vi "ECS-1408-FPGA2-EPTx.vi"() -> ()   [LabVIEW 2015, in "ECS-FPGA.lvlib"]
uses:
  ECS-FPGA.lvlib
  <vilib>/Powertrain Controls/Device Drivers/Engine Position Tracking/EPTx/RevA/FPGA/Controls/EPTxSupervisor.ctl
  <vilib>/Powertrain Controls/Device Drivers/Engine Position Tracking/EPTx/RevA/FPGA/Controls/EPTxFuelSparkControl.ctl
  <vilib>/Powertrain Controls/Device Drivers/Engine Position Tracking/EPTx/RevA/FPGA/Controls/EPTxControl.ctl
  <vilib>/Powertrain Controls/Device Drivers/Engine Position Tracking/EPTx/RevA/FPGA/Controls/EPTxConfig.ctl
  <vilib>/Powertrain Controls/Device Drivers/Engine Position Tracking/EPTx/RevA/FPGA/Controls/EPTxTooth.ctl
  <vilib>/Platform/TimedLoop/XDataNode/timing_clust.ctl
  <vilib>/Platform/TimedLoop/XDataNode/nitl_modes.ctl
  <vilib>/Platform/TimedLoop/XDataNode/wakeup.ctl
  <vilib>/Powertrain Controls/Device Drivers/Engine Position Tracking/EPTx/RevA/FPGA/Controls/EPTxSignals.ctl
  <vilib>/rvi/Emulation/niFpgaGetClockAttributes.vi
  <vilib>/rvi/Emulation/niFpgaSctlEmulationGetInTimedLoop.vi
  <vilib>/rvi/Emulation/niFpgaEmulationReportErrorSimple.vi
  <vilib>/rvi/eio/common/nirviEmuTemplateMethod_errors.vi
  <vilib>/rvi/Emulation/niFpgaCriticalErrorInLSC.vi
  <vilib>/eio/EIONode/EIONode.xnode
  <vilib>/Platform/TimedLoop/XDataNode/XDataNode.xnode
  <vilib>/Platform/TimedLoop/XDataNode/XDNodeRunTimeDep.lvlib
  <vilib>/Powertrain Controls/Device Drivers/Engine Position Tracking/EPTx/RevA/FPGA/EPTx - RevA - FPGA.lvlib
panel:
  in  "DI-4.PlsGen_Config_Channel3":T1
  in  "DI-4.PlsGen_Config_Channel2":T1
  in  "DI-4.PlsGen_Config_Channel1":T1
  in  "DI-3.PlsGen_Config_Channel3":T1
  in  "DI-3.PlsGen_Config_Channel2":T1
  in  "DI-3.PlsGen_Config_Channel1":T1
  in  "DI-2.PlsGen_Config_Channel3":T1
  in  "DI-2.PlsGen_Config_Channel2":T1
  in  "DI-2.PlsGen_Config_Channel1":T1
  out "EPTxTooth":T2
  in  "EPTxConfig":T3
  in  "EPTxControl":T4
  in  "9269-1.AO3":fxp<+/-,20,5> format="%.17g"
  in  "9269-1.AO2":fxp<+/-,20,5> format="%.17g"
  in  "9269-1.AO1":fxp<+/-,20,5> format="%.17g"
  in  "9269-1.AO0":fxp<+/-,20,5> format="%.17g"
  in  "ESTTL-1.Sequences":T5(array[cluster])
  in  "ESTTL-1.Config":T6
  in  "DI-4.Control":T7 caption="DIControl"
  in  "DI-4.IPhaseInterface":T8(array[cluster]) caption="IPhaseInterface"
  in  "DI-4.ScopeRead":bool caption="DIScopeRead"
  out "DI-4.ScopeData":T9 caption="DIScopeData"
  out "DI-4.Data":T10 caption="DIData"
  in  "DI-3.Control":T7 caption="DIControl"
  in  "DI-3.IPhaseInterface":T8(array[cluster]) caption="IPhaseInterface"
  in  "DI-3.ScopeRead":bool caption="DIScopeRead"
  out "DI-3.ScopeData":T9 caption="DIScopeData"
  out "DI-3.Data":T10 caption="DIData"
  in  "PFI-2.FuelControl 4":T11
  in  "PFI-2.FuelControl 3":T11
  in  "PFI-2.FuelControl 2":T11
  in  "PFI-2.FuelControl 1":T11
  out "EPTxSupervisor":T12
  out "DI-2.Data":T10 caption="DIData"
  out "PFI-2.Data":T13 caption="PFIData"
  in  "PFI-2.IPhaseInterface":T14(array[cluster])=[{"IPhaseCurrent"=0, "IPhaseDuration"=0}, {"IPhaseCurrent"=0, "IPhaseDuration"=0}, {"IPhaseCurrent"=0, "IPhaseDuration"=0}, {"IPhaseCurrent"=0, "IPhaseDuration"=0}, {"IPhaseCurrent"=0, "IPhaseDuration"=0}, {"IPhaseCurrent"=0, "IPhaseDuration"=0}, {"IPhaseCurrent"=0, "IPhaseDuration"=0}, {"IPhaseCurrent"=0, "IPhaseDuration"=0}] caption="IPhaseInterface"
  in  "PFI-2.LowsidePWM":T15 caption="LowsidePWM"
  in  "PFI-2.Control":T16 caption="PFIControl"
  out "DI-2.ScopeData":T9 caption="DIScopeData"
  in  "DI-2.ScopeRead":bool caption="DIScopeRead"
  in  "DI-2.IPhaseInterface":T8(array[cluster]) caption="IPhaseInterface"
  in  "DI-2.Control":T7 caption="DIControl"
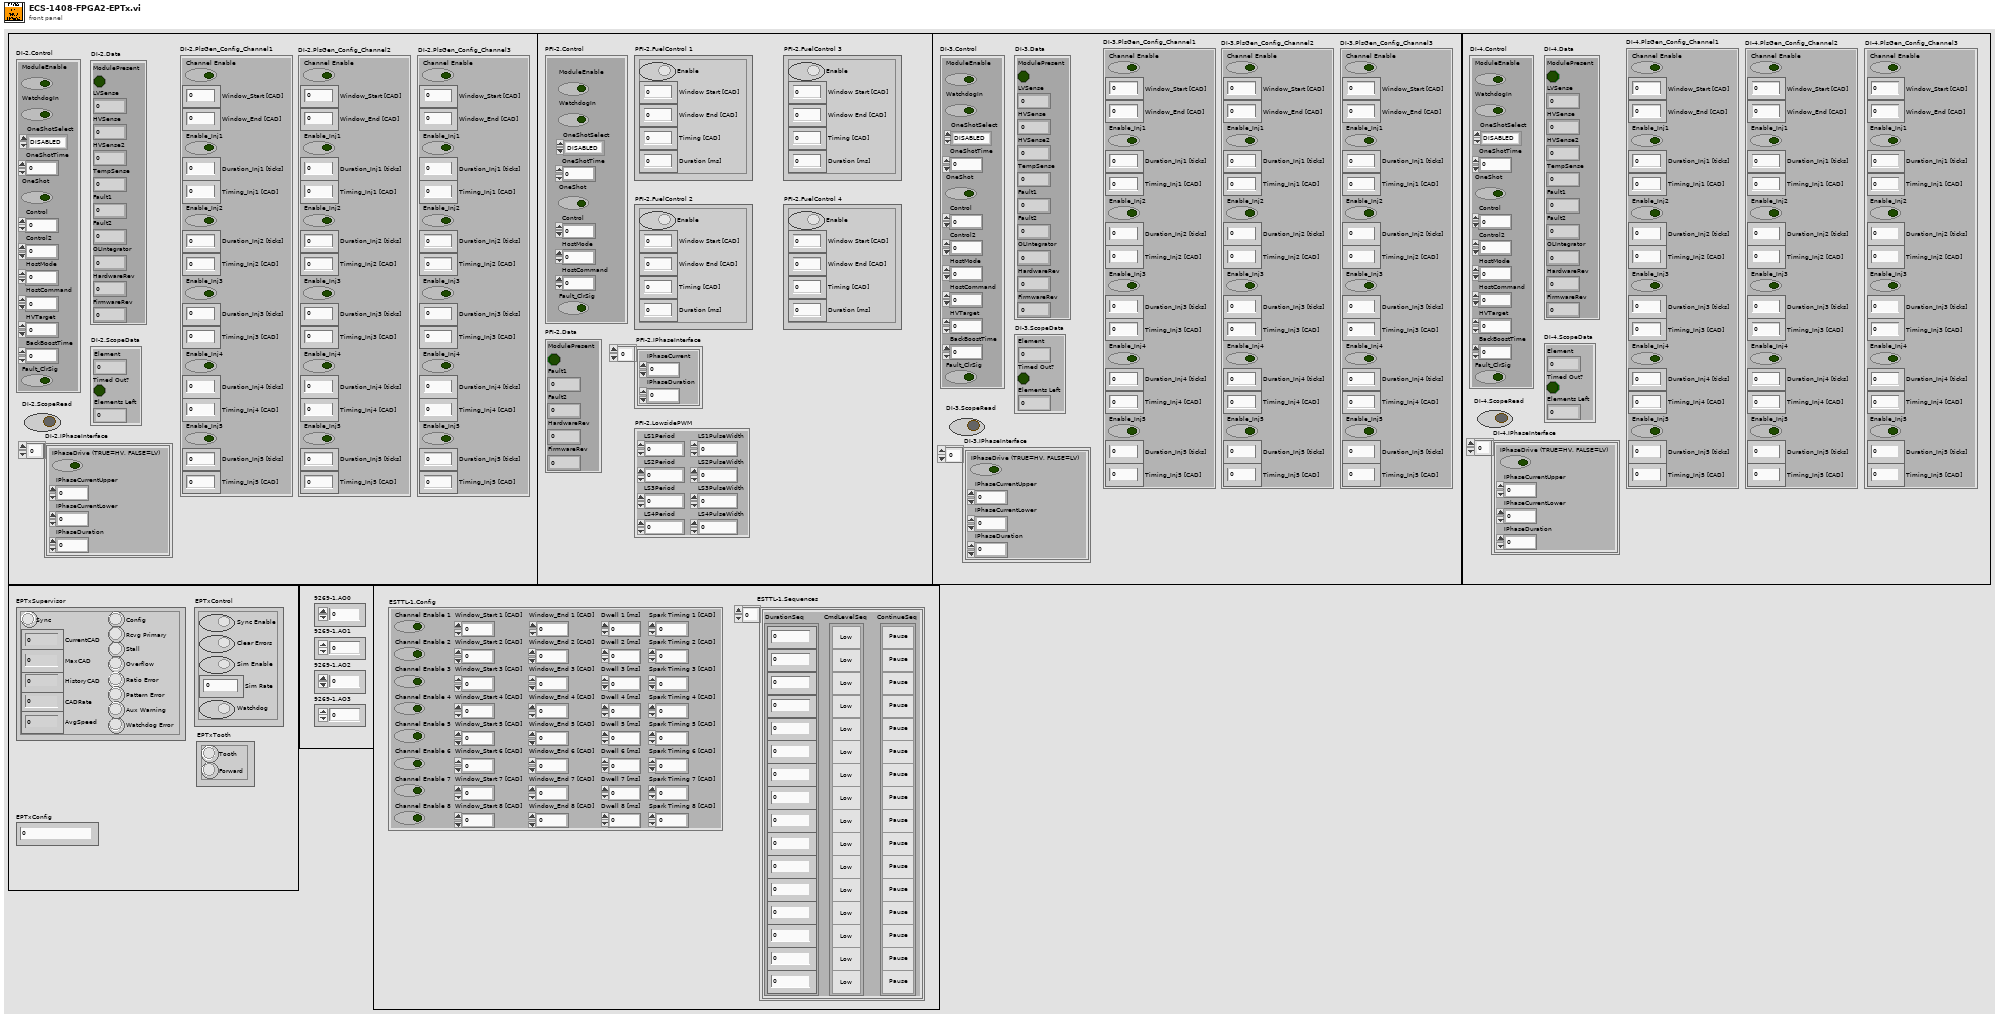
[diagram p1: front panel]
types:
  T1 = cluster{"Channel Enable":bool, "Window_Start [CAD]":fxp<+,18,11>, "Window_End [CAD]":fxp<+,18,11>, "Enable_Inj1":bool, "Duration_Inj1 [ticks]":u32, "Timing_Inj1 [CAD]":fxp<+,18,11>, "Enable_Inj2":bool, "Duration_Inj2 [ticks]":u32, "Timing_Inj2 [CAD]":fxp<+,18,11>, "Enable_Inj3":bool, "Duration_Inj3 [ticks]":u32, "Timing_Inj3 [CAD]":fxp<+,18,11>, "Enable_Inj4":bool, "Duration_Inj4 [ticks]":u32, "Timing_Inj4 [CAD]":fxp<+,18,11>, "Enable_Inj5":bool, "Duration_Inj5 [ticks]":u32, "Timing_Inj5 [CAD]":fxp<+,18,11>}
  T2 = typedef "EPTx - RevA - FPGA.lvlib/EPTxTooth.ctl" = cluster{"Tooth":bool, "Forward":bool}
  T3 = typedef "EPTx - RevA - FPGA.lvlib/EPTxConfig.ctl" = u64
  T4 = typedef "EPTx - RevA - FPGA.lvlib/EPTxControl.ctl" = cluster{"Sync Enable":bool, "Clear Errors":bool, "Sim Enable":bool, "Sim Rate":fxp<+,24,6>, "Watchdog":bool}
  T5 = cluster{"DurationSeq":u32[], "CmdLevelSeq":bool[], "ContinueSeq":bool[]}[]
  T6 = cluster{"Channel Enable 1":bool, "Window_Start 1 [CAD]":fxp<+,18,11>, "Window_End 1 [CAD]":fxp<+,18,11>, "Dwell 1 [ms]":fxp<+/-,22,9>, "Spark Timing 1 [CAD]":fxp<+,18,11>, "Channel Enable 2":bool, "Window_Start 2 [CAD]":fxp<+,18,11>, "Window_End 2 [CAD]":fxp<+,18,11>, "Dwell 2 [ms]":fxp<+/-,22,9>, "Spark Timing 2 [CAD]":fxp<+,18,11>, "Channel Enable 3":bool, "Window_Start 3 [CAD]":fxp<+,18,11>, "Window_End 3 [CAD]":fxp<+,18,11>, "Dwell 3 [ms]":fxp<+/-,22,9>, "Spark Timing 3 [CAD]":fxp<+,18,11>, "Channel Enable 4":bool, "Window_Start 4 [CAD]":fxp<+,18,11>, "Window_End 4 [CAD]":fxp<+,18,11>, "Dwell 4 [ms]":fxp<+/-,22,9>, "Spark Timing 4 [CAD]":fxp<+,18,11>, "Channel Enable 5":bool, "Window_Start 5 [CAD]":fxp<+,18,11>, "Window_End 5 [CAD]":fxp<+,18,11>, "Dwell 5 [ms]":fxp<+/-,22,9>, "Spark Timing 5 [CAD]":fxp<+,18,11>, "Channel Enable 6":bool, "Window_Start 6 [CAD]":fxp<+,18,11>, "Window_End 6 [CAD]":fxp<+,18,11>, "Dwell 6 [ms]":fxp<+/-,22,9>, "Spark Timing 6 [CAD]":fxp<+,18,11>, "Channel Enable 7":bool, "Window_Start 7 [CAD]":fxp<+,18,11>, "Window_End 7 [CAD]":fxp<+,18,11>, "Dwell 7 [ms]":fxp<+/-,22,9>, "Spark Timing 7 [CAD]":fxp<+,18,11>, "Channel Enable 8":bool, "Window_Start 8 [CAD]":fxp<+,18,11>, "Window_End 8 [CAD]":fxp<+,18,11>, "Dwell 8 [ms]":fxp<+/-,22,9>, "Spark Timing 8 [CAD]":fxp<+,18,11>}
  T7 = cluster{"ModuleEnable":bool, "WatchdogIn":bool, "OneShotSelect":enum8{"DISABLED", "CHAN 1", "CHAN 2", "CHAN 3"}, "OneShotTime":u32, "OneShot":bool, "Control":u8, "Control2":u8, "HostMode":u8, "HostCommand":u32, "HVTarget":u8, "BackBoostTime":u8, "Fault_ClrSig":bool}
  T8 = cluster{"IPhaseDrive (TRUE=HV, FALSE=LV)":bool, "IPhaseCurrentUpper":u16, "IPhaseCurrentLower":u16, "IPhaseDuration":u16}[]
  T9 = cluster{"Element":u32, "Timed Out?":bool, "Elements Left":u32}
  T10 = cluster{"ModulePresent":bool, "LVSense":u8, "HVSense":u8, "HVSense2":u8, "TempSense":i8, "Fault1":u8, "Fault2":u8, "OLIntegrator":u32, "HardwareRev":u8, "FirmwareRev":u8}
  T11 = typedef "EPTx - RevA - FPGA.lvlib/EPTxFuelSparkControl.ctl" = cluster{"Enable":bool, "Window Start [CAD]":fxp<+,18,11>, "Window End [CAD]":fxp<+,18,11>, "Timing [CAD]":fxp<+,18,11>, "Duration [ms]":fxp<+/-,22,9>}
  T12 = typedef "EPTx - RevA - FPGA.lvlib/EPTxSupervisor.ctl" = cluster{"Sync":bool, "CurrentCAD":fxp<+,18,11>, "MaxCAD":fxp<+,11,11>, "HistoryCAD":fxp<+,11,11>, "CADRate":fxp<+,22,8>, "AvgSpeed":fxp<+,17,15>, "Config":bool, "Rcvg Primary":bool, "Stall":bool, "Overflow":bool, "Ratio Error":bool, "Pattern Error":bool, "Aux Warning":bool, "Watchdog Error":bool}
  T13 = cluster{"ModulePresent":bool, "Fault1":u8, "Fault2":u8, "HardwareRev":u8, "FirmwareRev":u8}
  T14 = cluster{"IPhaseCurrent":u16, "IPhaseDuration":u16}[]
  T15 = cluster{"LS1Period":u32, "LS1PulseWidth":u32, "LS2Period":u32, "LS2PulseWidth":u32, "LS3Period":u32, "LS3PulseWidth":u32, "LS4Period":u32, "LS4PulseWidth":u32}
  T16 = cluster{"ModuleEnable":bool, "WatchdogIn":bool, "OneShotSelect":enum8{"DISABLED", "PFI 1", "PFI 2", "PFI 3", "PFI 4"}, "OneShotTime":u32, "OneShot":bool, "Control":u16, "HostMode":u8, "HostCommand":u32, "Fault_ClrSig":bool}
  T17 = typedef "XDNodeRunTimeDep.lvlib/timing_clust.ctl" = cluster{"Expected End [f-1]":u64, "Actual End [f-1]":u64, "Finished Late? [f-1]":bool, "Expected End [i-1]":u64, "Actual End [i-1]":u64, "Finished Late? [i-1]":bool, "Expected Start [i]":u64, "Actual Start [i]":u64, "Expected Start [f]":u64, "Actual Start [f]":u64, "Source Name":string, "Structure Name":string, "Period":i64, "Deadline":i64, "Offset":i64, "Start":i64, "Priority":i32, "Timeout":i32, "Mode":T18, "Wakeup Reason":T19, "Error":errorcluster, "Source Type":string, "Secondary Source Type":string, "Global End Time":u64, "Global Start Time":u64, "Frame Duration":u64, "Iteration Duration":u64, "Assigned CPU":i32, "I/O Scan Engine Mode":u32}
  T18 = typedef "XDNodeRunTimeDep.lvlib/nitl_modes.ctl" = enum32{"No Change", "Process missed periods, maintain original phase", "Discard missed periods, maintain original phase", "Process missed periods, ignore original phase", "Discard missed periods, ignore original phase"}
  T19 = typedef "XDNodeRunTimeDep.lvlib/wakeup.ctl" = enum32{"Normal", "Aborted", "Asynchronous wakeup", "Timing source error", "Timed loop error", "Timeout"}
  T20 = typedef "EPTx - RevA - FPGA.lvlib/EPTxSignals.ctl" = cluster{"Primary":bool, "Aux 1":bool, "Aux 2":bool, "Aux 3":bool, "Aux 4":bool}
  T21 = cluster{"CmdOut1":bool, "CmdOut2":bool, "CmdOut3":bool, "CmdOut4":bool, "CmdOut5":bool, "CmdOut6":bool, "CmdOut7":bool, "CmdOut8":bool}
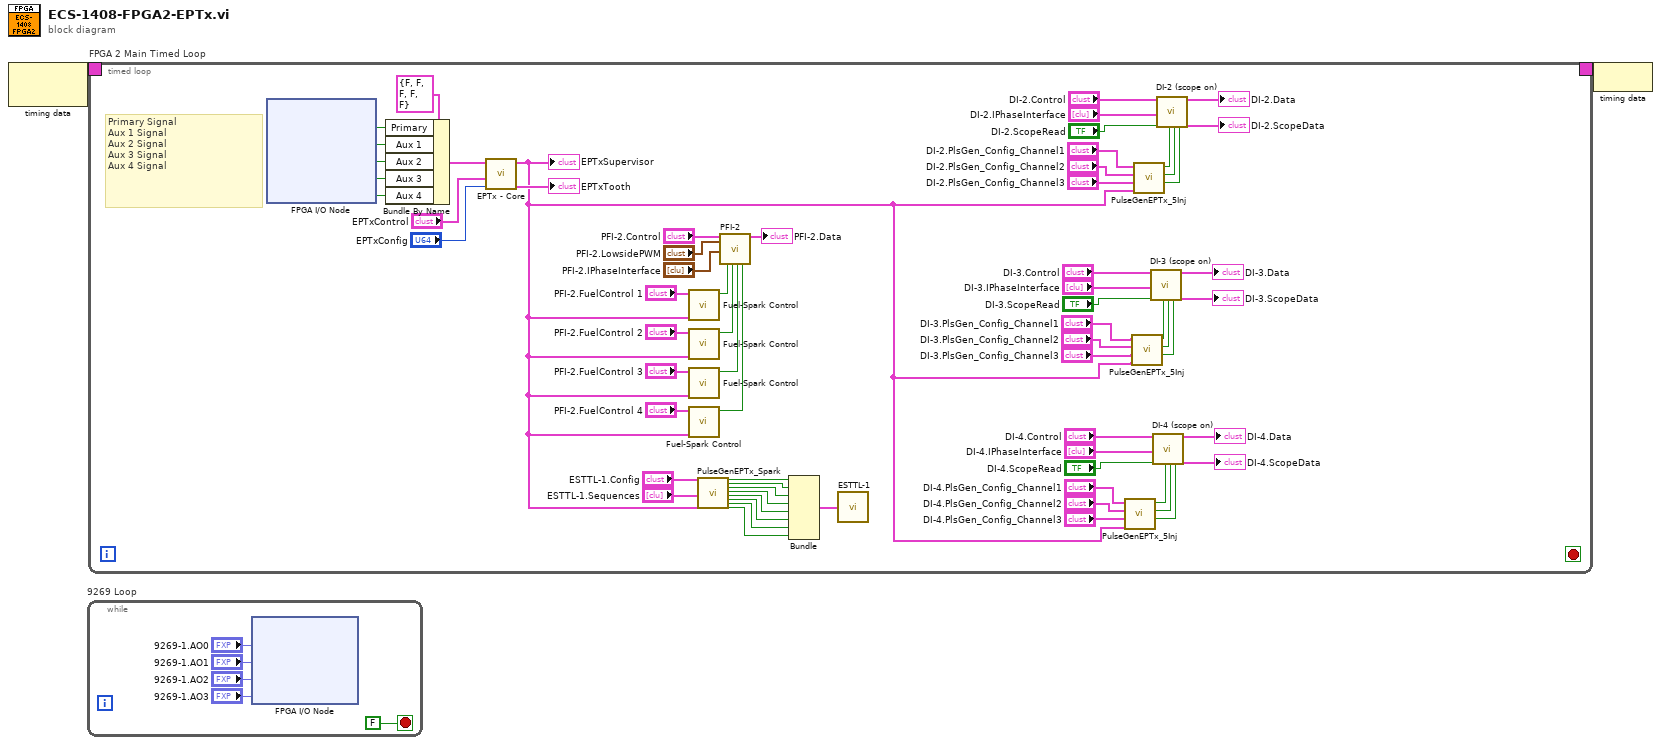
[diagram p0: block diagram]
diagram:
  n1 = node-c288() -> (w2:T17)  [unwired: 1 in]
  n2 = while "9269 Loop" {
    stop <- FALSE stop-if-true
    n3 = xnode "FPGA I/O Node"("9269-1/AO0"="9269-1.AO0", "9269-1/AO1"="9269-1.AO1", "9269-1/AO2"="9269-1.AO2", "9269-1/AO3"="9269-1.AO3") -> ()  [unwired: 4 in, 4 out]
  }
  n4 = timed-loop "FPGA 2 Main Timed Loop" {
    timing: w2 -> [_]
    timing-out: [_] -> w1
    stop <- _ stop-if-true
    # "Primary Signal\nAux 1 Signal\nAux 2 Signal\nAux 3 Signal\nAux 4 Signal"
    n5 = xnode "FPGA I/O Node"() -> ("9401-2/DIO2"=w38:bool, "9401-2/DIO3"=w37:bool, "9401-2/DIO4"=w36:bool, "9401-2/DIO5"=w35:bool, "9401-2/DIO6"=w34:bool)  [unwired: 5 in, 5 out]
    n6 = Bundle By Name(cluster=T20 {"Primary"=FALSE, "Aux 1"=FALSE, "Aux 2"=FALSE, "Aux 3"=FALSE, "Aux 4"=FALSE} ("EPTxSignals"), "Primary"=w38, "Aux 1"=w37, "Aux 2"=w36, "Aux 3"=w35, "Aux 4"=w34) -> (w39:T20)
    n7 = call <vilib>:"EPTx - Core.vi"("EPTxConfig"="EPTxConfig", "EPTxControl"="EPTxControl", "EPTxSignals"=w39) -> ("EPTxTooth"=→"EPTxTooth":T2, "EPTxSupervisor"=w17:T12)  [unwired: 7 in]
    "EPTxSupervisor" <- w17
    n8 = call <vilib>:"Fuel-Spark Control.vi"("EPTxSupervisor"=w17, "Fuel-Spark Control"="PFI-2.FuelControl 1") -> ("Fuel-Spark Command"=w60:bool)  [unwired: 9 in]
    n9 = call <vilib>:"Fuel-Spark Control.vi"("EPTxSupervisor"=w17, "Fuel-Spark Control"="PFI-2.FuelControl 2") -> ("Fuel-Spark Command"=w61:bool)  [unwired: 9 in]
    n10 = call <vilib>:"Fuel-Spark Control.vi"("EPTxSupervisor"=w17, "Fuel-Spark Control"="PFI-2.FuelControl 3") -> ("Fuel-Spark Command"=w62:bool)  [unwired: 9 in]
    n11 = call <vilib>:"Fuel-Spark Control.vi"("EPTxSupervisor"=w17, "Fuel-Spark Control"="PFI-2.FuelControl 4") -> ("Fuel-Spark Command"=w63:bool)  [unwired: 9 in]
    n12 = call "PulseGenEPTx_Spark.vi"("Spark_Config"="ESTTL-1.Config", "Spark_Sequences"="ESTTL-1.Sequences", "EPTxSupervisor"=w17) -> ("CmdOut1"=w51:bool, "CmdOut2"=w50:bool, "CmdOut3"=w49:bool, "CmdOut4"=w48:bool, "CmdOut5"=w47:bool, "CmdOut6"=w46:bool, "CmdOut7"=w45:bool, "CmdOut8"=w44:bool)  [unwired: 17 in]
    n13 = call "PFI-2"("PFI-2_Control"="PFI-2.Control", "PFI-2_LowsidePWM"="PFI-2.LowsidePWM", "PFI-2_IPhaseInterface"="PFI-2.IPhaseInterface", "PFI1Cmd"=w60, "PFI2Cmd"=w61, "PFI3Cmd"=w62, "PFI4Cmd"=w63) -> ("PFI-2_Data"=→"PFI-2.Data":T13)  [unwired: 11 in, 1 out]
    n14 = Bundle("CmdOut1"=w51, "CmdOut2"=w50, "CmdOut3"=w49, "CmdOut4"=w48, "CmdOut5"=w47, "CmdOut6"=w46, "CmdOut7"=w45, "CmdOut8"=w44) -> (w43:T21)  [unwired: 1 out]
    n15 = call "ESTTL-1"("ESTTL-1_ESTTLChan"=w43) -> ()  [unwired: 1 out]
    n16 = call "PulseGenEPTx_5Inj.vi"("EPTxSupervisor"=w17, "Inj_Config_Channel3"="DI-4.PlsGen_Config_Channel3", "Inj_Config_Channel2"="DI-4.PlsGen_Config_Channel2", "Inj_Config_Channel1"="DI-4.PlsGen_Config_Channel1") -> ("CmdOut3"=w14:bool, "CmdOut2"=w15:bool, "CmdOut1"=w16:bool)  [unwired: 3 in]
    n17 = call "PulseGenEPTx_5Inj.vi"("EPTxSupervisor"=w17, "Inj_Config_Channel3"="DI-3.PlsGen_Config_Channel3", "Inj_Config_Channel2"="DI-3.PlsGen_Config_Channel2", "Inj_Config_Channel1"="DI-3.PlsGen_Config_Channel1") -> ("CmdOut3"=w21:bool, "CmdOut2"=w22:bool, "CmdOut1"=w23:bool)  [unwired: 3 in]
    n18 = call "PulseGenEPTx_5Inj.vi"("EPTxSupervisor"=w17, "Inj_Config_Channel3"="DI-2.PlsGen_Config_Channel3", "Inj_Config_Channel2"="DI-2.PlsGen_Config_Channel2", "Inj_Config_Channel1"="DI-2.PlsGen_Config_Channel1") -> ("CmdOut3"=w27:bool, "CmdOut2"=w10:bool, "CmdOut1"=w11:bool)  [unwired: 3 in]
    n19 = call "DI-3 (scope on)"("DI-3_Control"="DI-3.Control", "DI-3_IPhaseInterface"="DI-3.IPhaseInterface", "DI-3_ScopeRead"="DI-3.ScopeRead", "DI1Cmd"=w23, "DI2Cmd"=w22, "DI3Cmd"=w21) -> ("DI-3_Data"=→"DI-3.Data":T10, "DI-3_ScopeData"=→"DI-3.ScopeData":T9)  [unwired: 11 in, 1 out]
    n20 = call "DI-4 (scope on)"("DI-4_Control"="DI-4.Control", "DI-4_IPhaseInterface"="DI-4.IPhaseInterface", "DI-4_ScopeRead"="DI-4.ScopeRead", "DI1Cmd"=w16, "DI2Cmd"=w15, "DI3Cmd"=w14) -> ("DI-4_Data"=→"DI-4.Data":T10, "DI-4_ScopeData"=→"DI-4.ScopeData":T9)  [unwired: 11 in, 1 out]
    n21 = call "DI-2 (scope on)"("DI-2_Control"="DI-2.Control", "DI-2_IPhaseInterface"="DI-2.IPhaseInterface", "DI-2_ScopeRead"="DI-2.ScopeRead", "DI1Cmd"=w11, "DI2Cmd"=w10, "DI3Cmd"=w27) -> ("DI-2_Data"=→"DI-2.Data":T10, "DI-2_ScopeData"=→"DI-2.ScopeData":T9)  [unwired: 11 in, 1 out]
  }
  n22 = node-c288(w1) -> ()
